vi "Append AxialScan(MC).vi"(9 "Reference Data":T1={"Refrence data path"=path "", "Reference Rectangle"=[], "AOL Z"=0.0, "No of pixels in a miniscan "=[], "Threshold"=[], "No of miniscans"=[], "Full Frame Size"=0, "Reference Image"=refnum, "dwelltime"=0.1, "Zoom"=1.0, "Field of View"=0.0, "Z Step"=1, "Z pixels"=1, "Z Lines"=1, "Z Ignore"=1, "Laser"=1}, 11 "miniScan_Coordinates":T3) -> (3 "miniScan_Coordinates":T3)   [LabVIEW 2020]
uses:
  Typedefs/Reference_Globals.ctl
  <vilib>/vision/Image Controls.llb/IMAQ Image.ctl
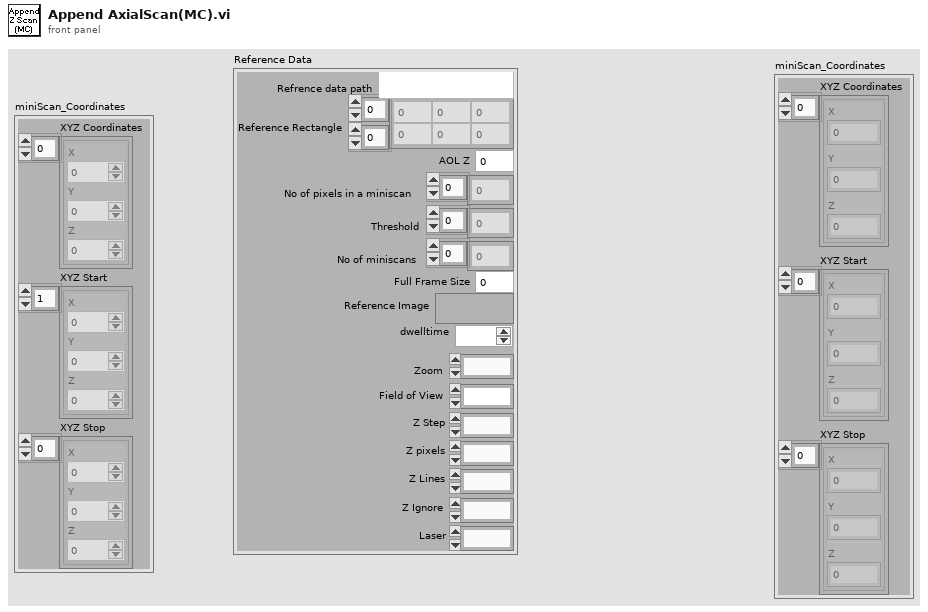
[diagram p1: front panel]
types:
  T1 = typedef "Reference_Globals.ctl" = cluster{"Refrence data path":path, "Reference Rectangle":i16[][], "AOL Z":dbl, "No of pixels in a miniscan ":i32[], "Threshold":i16[], "No of miniscans":i32[], "Full Frame Size":u16, "Reference Image":T2, "dwelltime":dbl, "Zoom":dbl, "Field of View":dbl, "Z Step":i8, "Z pixels":i32, "Z Lines":u8, "Z Ignore":u8, "Laser":u8}
  T2 = typedef "IMAQ Image.ctl" = refnum<image>
  T3 = cluster{"XYZ Coordinates":cluster{"X":sgl, "Y":sgl, "Z":sgl}[], "XYZ Start":cluster{"X":dbl, "Y":dbl, "Z":dbl}[], "XYZ Stop":cluster{"X":dbl, "Y":dbl, "Z":dbl}[]}
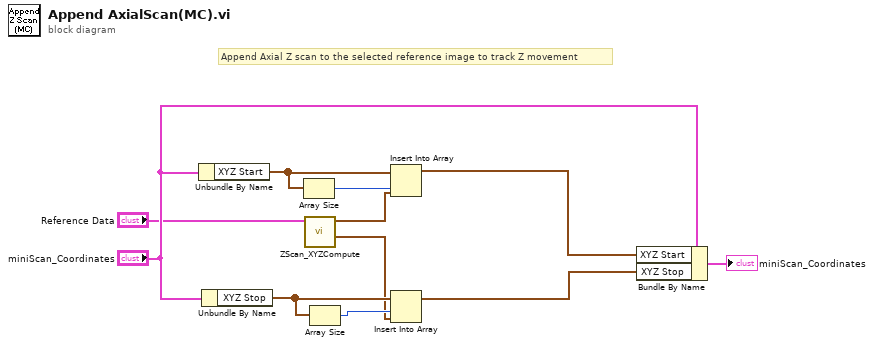
[diagram p0: block diagram]
diagram:
  # "Append Axial Z scan to the selected reference image to track Z movement"
  n1 = Unbundle By Name("miniScan_Coordinates") -> ("XYZ Start"=w11:cluster{"X":dbl, "Y":dbl, "Z":dbl}[])
  n2 = Unbundle By Name("miniScan_Coordinates") -> ("XYZ Stop"=w5:cluster{"X":dbl, "Y":dbl, "Z":dbl}[])
  n3 = Array Size(array=w11) -> (size(s)=w10:i32)
  n4 = call "ZScan_XYZCompute.vi"("Reference Data"="Reference Data") -> ("XYZ Stop"=w1:cluster{"X":dbl, "Y":dbl, "Z":dbl}[], "XYZ Start"=w2:cluster{"X":dbl, "Y":dbl, "Z":dbl}[])  [unwired: 9 in]
  n5 = Array Size(array=w5) -> (size(s)=w4:i32)
  n6 = Insert Into Array(array=w11, index=w10, new element=w2) -> (w8:cluster{"X":dbl, "Y":dbl, "Z":dbl}[])
  n7 = Insert Into Array(array=w5, index=w4, new element=w1) -> (w7:cluster{"X":dbl, "Y":dbl, "Z":dbl}[])
  n8 = Bundle By Name(cluster="miniScan_Coordinates", "XYZ Start"=w8, "XYZ Stop"=w7) -> (→"miniScan_Coordinates":T3)
